vi "Set EOF String.vi"(8 "error in (no error)":errorcluster, 9 "2nd Character (0)":i32, 10 "1st Character (0)":i32, 11 "VISA resource name":refnum<visa-resource-name>) -> (0 "error out":errorcluster, 3 "VISA resource name out":refnum<visa-resource-name>)   [LabVIEW 2013, in "Fluke 5XXX Series Multicalibrators.lvlib"]
doc: "This VI sets the End-Of-File character string for the RS-232-C serial interface. The EOF setting is saved when the power is turned off.\n\nNote:\n\nThis VI is available only for instrument models 5700A and 5720A."
uses:
  Fluke 5XXX Series Multicalibrators.lvlib
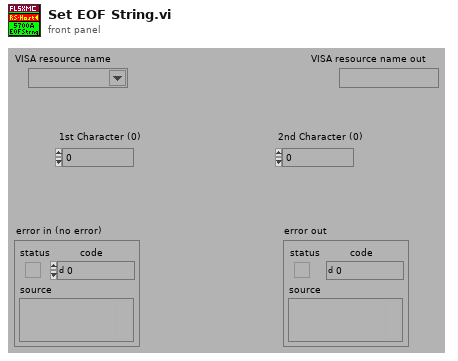
[diagram p1: front panel]
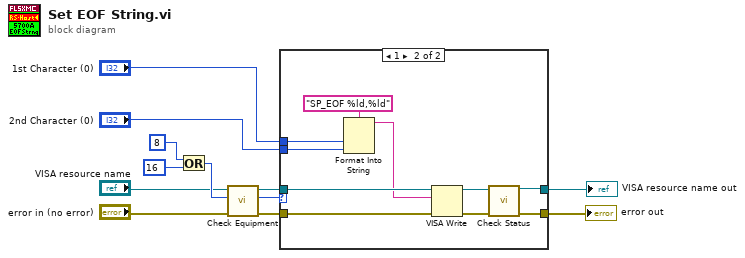
[diagram p0: block diagram]
diagram:
  n1 = Or(x=8 ("Numeric"), y=16 ("Numeric")) -> (x .or. y?=w7:i32)
  n2 = call "Check Equipment.vi"("error in (no error)"="error in (no error)", "Bit Mask"=w7, "VISA resource name"="VISA resource name") -> ("error out"=w12:errorcluster, "Present?"=w11:u32, "VISA resource name out"=w10:refnum<visa-resource-name>)  [unwired: 6 in]
  n3 = case shown="1" w11 {
    tunnel: [w13 w21] -> w5
    tunnel: w12 -> [w14 w24]
    tunnel: w10 -> [w13 w23]
    tunnel: [w14 w22] -> w6
    tunnel: "2nd Character (0)" -> [_ w16]
    tunnel: "1st Character (0)" -> [_ w15]
    frame 0, Default {
    }
    frame 1 {
      n4 = Format Into String(format string="SP_EOF %ld,%ld", w15, w16) -> (resulting string=w17:string)  [unwired: 2 in, 1 out]
      n5 = VISA Write(VISA resource name=w23, write buffer=w17, error in (no error)=w24) -> (VISA resource name out=w20:refnum<visa-resource-name>, error out=w19:errorcluster)  [unwired: 1 out]
      n6 = call "Check Status.vi"("VISA resource name"=w20, "error in (no error)"=w19) -> ("VISA resource name out"=w21:refnum<visa-resource-name>, "error out"=w22:errorcluster)  [unwired: 12 in]
    }
  }
  "VISA resource name out" <- w5
  "error out" <- w6
